vi "Do.vi"(8 "error in (no error)":errorcluster, 10 "Actor in":refnum<class "Simple Actor.lvclass">, 11 "Initialize Msg in":refnum<class "Initialize Msg.lvclass">) -> (0 "error out":errorcluster, 2 "Actor out":refnum<class "Simple Actor.lvclass">, 3 "Initialize Msg out":refnum<class "Initialize Msg.lvclass">)   [LabVIEW 2020, in "Simple Actor.lvlib" / "Initialize Msg.lvclass"]
uses:
  Initialize Msg.lvclass
  Simple Actor/Simple Actor.lvclass
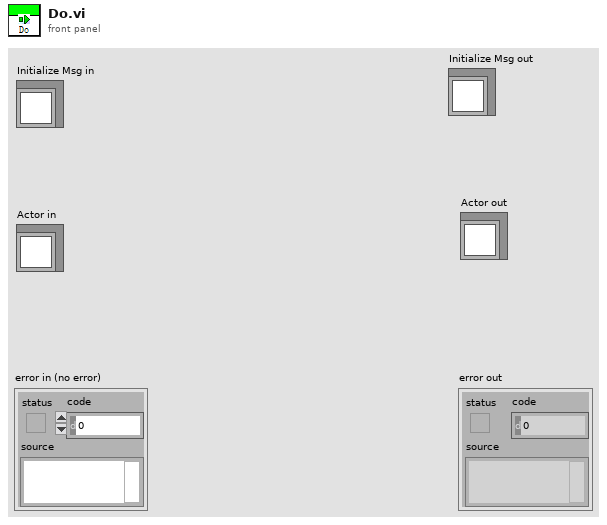
[diagram p1: front panel]
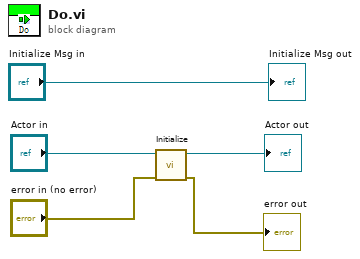
[diagram p0: block diagram]
diagram:
  n1 = call "Initialize.vi"("error in (no error)"="error in (no error)", "Simple Actor in"="Actor in") -> ("error out"=→"error out":errorcluster, "Simple Actor out"=→"Actor out":refnum<class "Simple Actor.lvclass">)  [unwired: 8 in]
  "Initialize Msg out" <- "Initialize Msg in"
